vi "DualFrequencySegments.vi"(9 "High Frequency IN":dbl=80000000.0, 11 "Low Frequency":dbl=100000.0) -> (1 "N rep High":dbl, 2 "Nhigh":dbl, 3 "N points":i32, 6 "sample rate (Hz)":dbl)   [LabVIEW 2015, in "ArbitraryFunctions.lvlib"]
uses:
  ArbitraryFunctions.lvlib
panel:
  out "Low Frequency OUT":dbl=100000.0
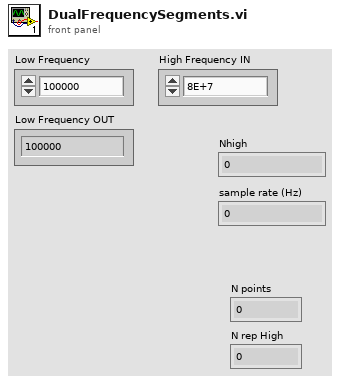
[diagram p1: front panel]
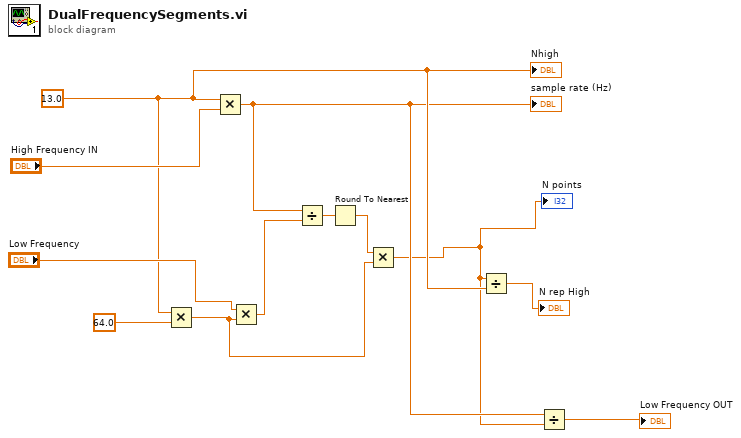
[diagram p0: block diagram]
diagram:
  w5 = 13.0 ("x")
  n1 = Multiply(x=w5, y=64.0 ("x")) -> (x*y=w4:dbl)
  n2 = Multiply(x=w5, y="High Frequency IN") -> (x*y=w3:dbl)
  "sample rate (Hz)" <- w3
  n3 = Multiply(x="Low Frequency", y=w4) -> (x*y=w9:dbl)
  n4 = Divide(x=w3, y=w9) -> (x/y=w11:dbl)
  n5 = Round To Nearest(number=w11) -> (nearest integer value=w8:dbl)
  n6 = Multiply(x=w8, y=w4) -> (x*y=w2:dbl)
  "N points" <- w2
  n7 = Divide(x=w2, y=w5) -> (x/y=→"N rep High":dbl)
  n8 = Divide(x=w3, y=w2) -> (x/y=→"Low Frequency OUT":dbl)
  "Nhigh" <- w5
